vi "Set King Position.vi"(0 "Input Parsed.King":T1, 11 "error in (no error)":errorcluster) -> (4 "King Set Output":string, 15 "error out":errorcluster)   [LabVIEW 2014, in "Dragon Tamers.lvlib"]
uses:
  Dragon Tamers.lvlib
  Typedefs/King.ctl
  Typedefs/Cell Pos.ctl
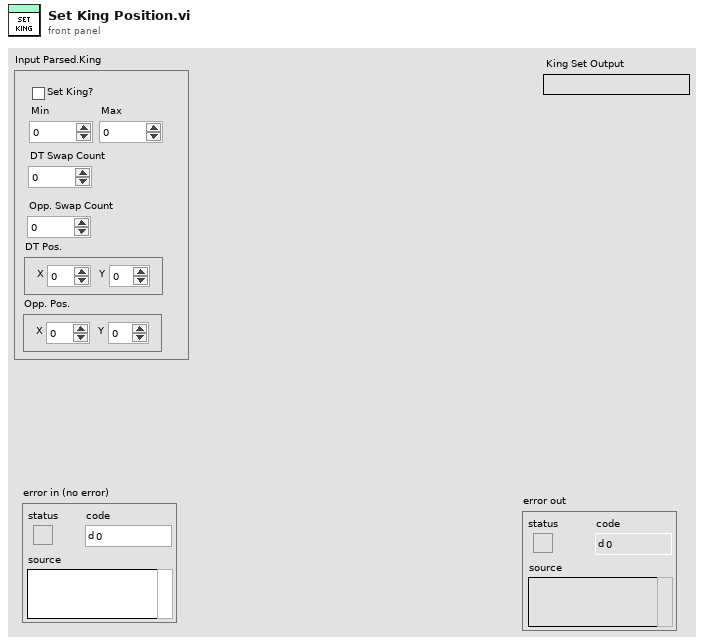
[diagram p1: front panel]
types:
  T1 = typedef "Dragon Tamers.lvlib/King.ctl" = cluster{"Set King?":bool, "Min":i32, "Max":i32, "DT Swap Count":i32, "Opp. Swap Count":i32, "DT Pos.":T2, "Opp. Pos.":T2}
  T2 = typedef "Dragon Tamers.lvlib/Cell Pos.ctl" = cluster{"X":i32, "Y":i32}
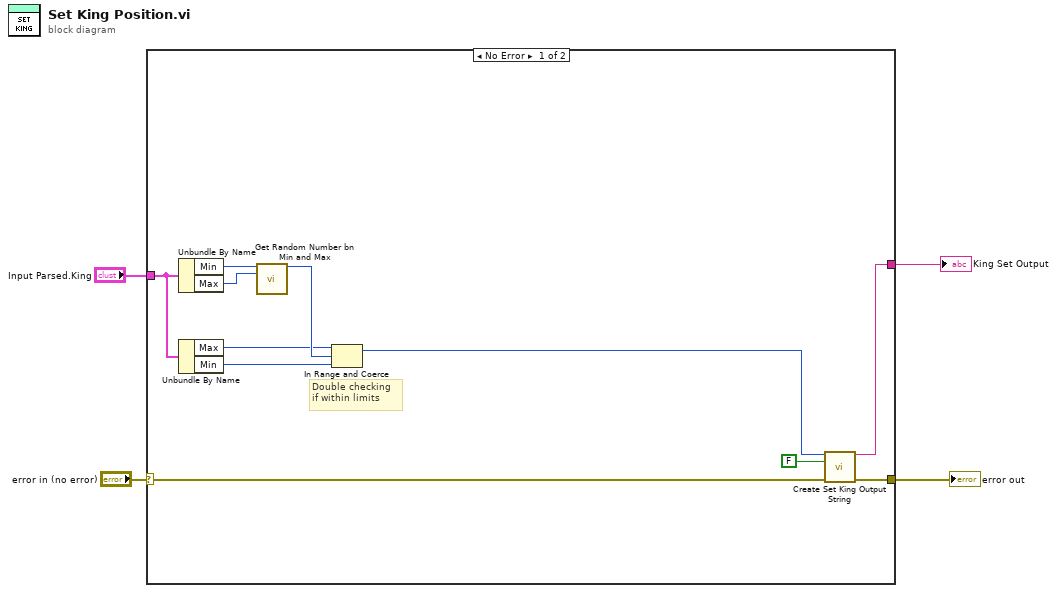
[diagram p0: block diagram]
diagram:
  n1 = case shown="No Error" "error in (no error)" {
    selector: "error in (no error)" -> [w9 w16]
    tunnel: [w8 w16] -> w3
    tunnel: "Input Parsed.King" -> [w12 _]
    tunnel: [w5 _] -> w1
    frame No Error {
      # "Double checking\nif within limits"
      n2 = Unbundle By Name(w12) -> ("Min"=w15:i32, "Max"=w14:i32)
      n3 = Unbundle By Name(w12) -> ("Max"=w11:i32, "Min"=w10:i32)
      n4 = call "Get Random Number bn Min and Max.vi"("Min"=w15, "Max"=w14) -> ("Random Value"=w13:i32)  [unwired: 13 in]
      n5 = In Range and Coerce(upper limit=w11, x=w13, lower limit=w10) -> (coerced(x)=w6:i32)  [unwired: 1 out]
      n6 = call "Create Set King Output String.vi"("Cell Index"=w6, "Zero Indexed? (T)"=FALSE, "error in (no error)"=w9) -> ("Output Text"=w5:string, "error out"=w8:errorcluster)  [unwired: 11 in]
    }
    frame Error {
    }
  }
  "error out" <- w3
  "King Set Output" <- w1
